vi "XML.InsertRootNode.vi"(8 "error in (no error)":errorcluster, 10 "Root name":string="HWConfigFile", 11 "doc":u32) -> (0 "error out":errorcluster, 2 "node out":u32, 3 "doc out":u32)   [LabVIEW 2019, in "Tools.lvlib"]
uses:
  Tools.lvlib
  LibXML/LibXML.lvlib
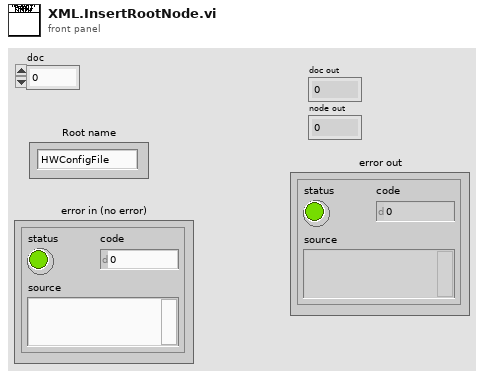
[diagram p1: front panel]
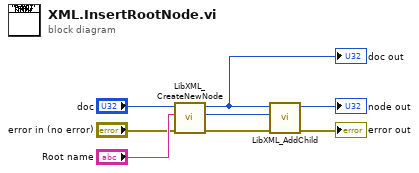
[diagram p0: block diagram]
diagram:
  n1 = call "LibXML_CreateNewNode.vi"("error in"="error in (no error)", "name"="Root name", "doc"="doc") -> ("error out"=w5:errorcluster, "nodePtr out"=w3:u32, "doc out"=w4:u32)  [unwired: 6 in]
  "doc out" <- w4
  n2 = call "LibXML_AddChild.vi"("error in"=w5, "parent"=w3, "node"=w4) -> ("error out"=→"error out":errorcluster, "node copy"=→"node out":u32)  [unwired: 7 in]
